vi "Settings - Default.vi"(8 "Error In":errorcluster, 11 "Module Name In":string) -> (0 "Error Out":errorcluster={"status"=TRUE, "code"=-200077, "source"="Property Node DAQmx Channel (arg 2) in DAQmx Create Channel (AI-Temperature-Thermocouple).vi:1->Settings - NI 9211.vi <append>\n<B>Property: </B>AI.Temp.Units\n<B>Requested Value: </B>\n<B>You Can Select: </B>Deg C, Deg F, Kelvins, Deg R, From Custom Scale\n\n<B>Channel Name: </B>Temperature\n\n<B>Task Name: </B>_unnamedTask<E>"}, 3 "Cancelled?":bool)   [LabVIEW 2011]
doc: "This VI will be launched for modules that are not yet supported (no settings VI ready)"
panel:
  in  "Cancel Button":bool
  in  "OK Button":bool
  out "MSG":string
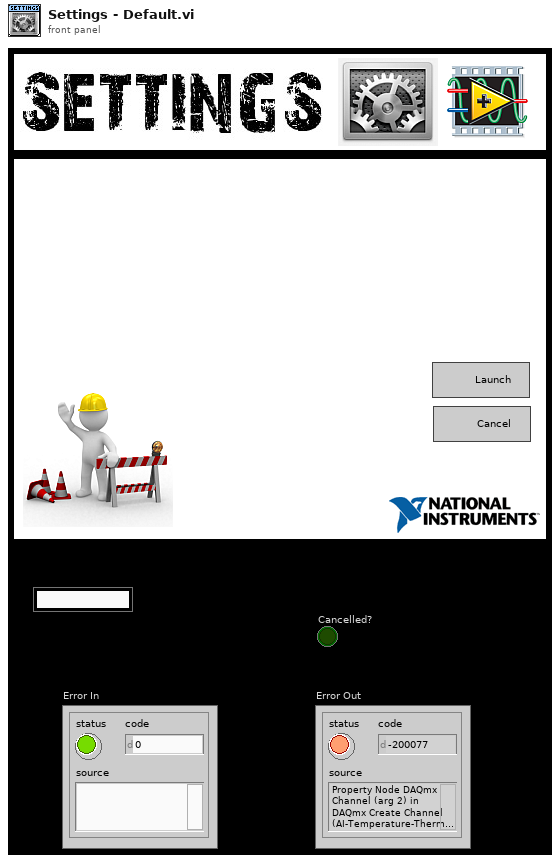
[diagram p1: front panel]
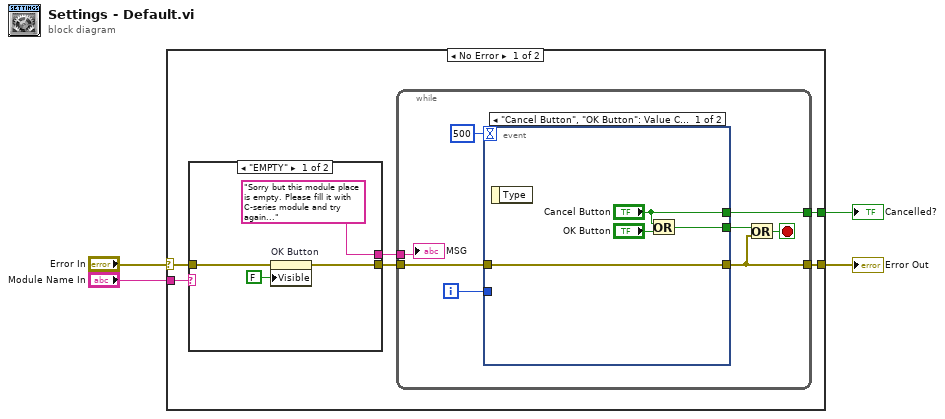
[diagram p0: block diagram]
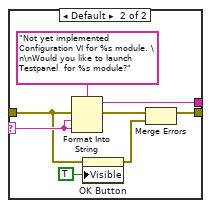
[diagram p2: hidden frame]
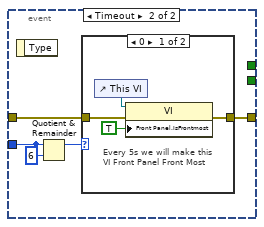
[diagram p3: hidden frame]
diagram:
  n1 = case shown="No Error" "Error In" {
    selector: "Error In" -> [w7 w44]
    tunnel: "Module Name In" -> [w5 _]
    tunnel: [w8 w44] -> w3
    tunnel: [w6 _] -> w1
    frame No Error {
      n2 = case shown="\"EMPTY\"" w5 {
        selector: w5 -> [_ w20]
        tunnel: ["Sorry but this module place is empty. Please fill it with C-series module and try again..." w21] -> w10
        tunnel: [w12 w18] -> w9
        tunnel: w7 -> [w13 w16]
        frame "EMPTY" {
          n3 = property on="OK Button" class="Bool"(error in=w13, "Visible"=FALSE) -> (error out=w12:errorcluster)  [unwired: 1 in, 1 out]
        }
        frame Default {
          n4 = Format Into String(format string="Not yet implemented Configuration VI for %s module. \n\nWould you like to launch Testpanel  for %s module?", error in=w16, w20, w20) -> (resulting string=w21:string, error out=w19:errorcluster)  [unwired: 1 in]
          n5 = property on="OK Button" class="Bool"(error in=w16, "Visible"=TRUE) -> (error out=w15:errorcluster)  [unwired: 1 in, 1 out]
          n6 = Merge Errors(w19, w15) -> (w18:errorcluster)
        }
      }
      n7 = while {
        tunnel: w9 -> [w30]
        tunnel: w10 -> [w29]
        tunnel: [w28] -> w8
        tunnel: [w25] -> w6
        i -> [w24]
        stop <- w26 stop-if-true
        n8 = event shown="[0] \"Cancel Button\", \"OK Button\": Value Change" {
          selector: _ -> [_ _]
          dyn-events: _ -> [_ _]
          timeout: 500 -> [_ _]
          tunnel: w30 -> [w34 w39]
          tunnel: [w34 w38] -> w28
          tunnel: [w32 _] -> w27
          tunnel: ["Cancel Button" _] -> w25
          tunnel: [_ w37] -> _
          tunnel: w24 -> [_ w37]
          event "Cancel Button", "OK Button": Value Change {
            n9 = event-data() -> ()  [unwired: 1 in, 1 out]
            n10 = Or(x="Cancel Button", y="OK Button") -> (x .or. y?=w32:bool)
          }
          event Timeout {
            n11 = event-data() -> ()  [unwired: 1 in, 1 out]
            n12 = Quotient & Remainder(x=w37, y=6) -> (x-y*floor(x/y)=w35:i32)  [unwired: 1 out]
            n13 = case shown="0" w35 {
              tunnel: w39 -> [w42 w43]
              tunnel: [w42 w43] -> w38
              frame 0 {
                # "Every 5s we will make this\nVI Front Panel Front Most"
                n14 = control-ref of="This VI"() -> (w41:refnum<vi>)
                n15 = property class="VI"(reference=w41, "Front Panel.IsFrontmost"=TRUE ("Front Panel Window:Is Frontmost")) -> ()  [unwired: 1 in, 2 out]
              }
              frame Default {
              }
            }
          }
        }
        n16 = Or(x=w27, y=w28) -> (x .or. y?=w26:bool)
        "MSG" <- w29
      }
    }
    frame Error {
    }
  }
  "Cancelled?" <- w1
  "Error Out" <- w3
